vi "HEWH Pressure Calculation.vi"(9 "MW100 Data Cluster":T1) -> (1 "Pressure Adjusted":T1)   [LabVIEW 2019]
uses:
  Type Definitions/HEWH MW100 Data Cluster.ctl
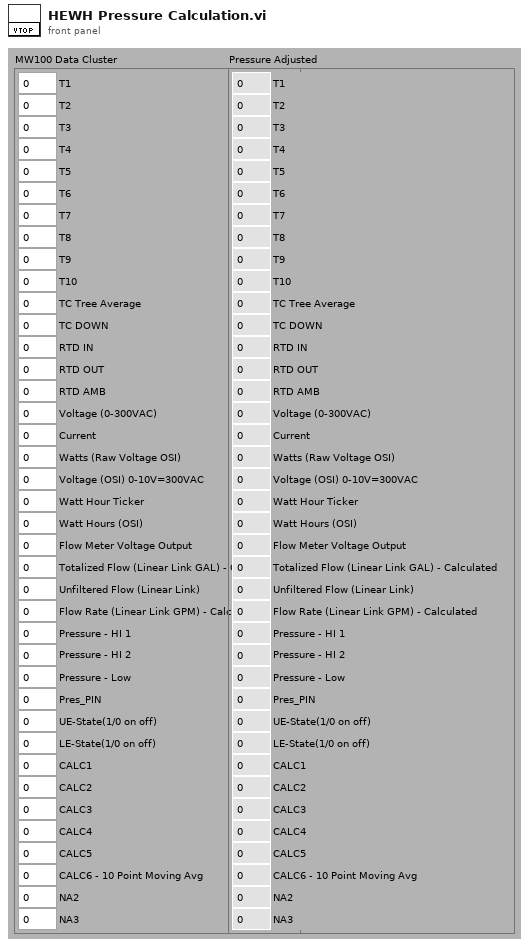
[diagram p1: front panel]
types:
  T1 = typedef "HEWH MW100 Data Cluster.ctl" = cluster{"T1":dbl, "T2":dbl, "T3":dbl, "T4":dbl, "T5":dbl, "T6":dbl, "T7":dbl, "T8":dbl, "T9":dbl, "T10":dbl, "TC Tree Average":dbl, "TC DOWN":dbl, "RTD IN":dbl, "RTD OUT":dbl, "RTD AMB":dbl, "Voltage (0-300VAC)":dbl, "Current":dbl, "Watts (Raw Voltage OSI)":dbl, "Voltage (OSI) 0-10V=300VAC":dbl, "Watt Hour Ticker":dbl, "Watt Hours (OSI)":dbl, "Flow Meter Voltage Output":dbl, "Totalized Flow (Linear Link GAL) - Calculated":dbl, "Unfiltered Flow (Linear Link)":dbl, "Flow Rate (Linear Link GPM) - Calculated":dbl, "Pressure - HI 1":dbl, "Pressure - HI 2":dbl, "Pressure - Low":dbl, "Pres_PIN":dbl, "UE-State(1/0 on off)":dbl, "LE-State(1/0 on off)":dbl, "CALC1":dbl, "CALC2":dbl, "CALC3":dbl, "CALC4":dbl, "CALC5":dbl, "CALC6 - 10 Point Moving Avg":dbl, "NA2":dbl, "NA3":dbl}
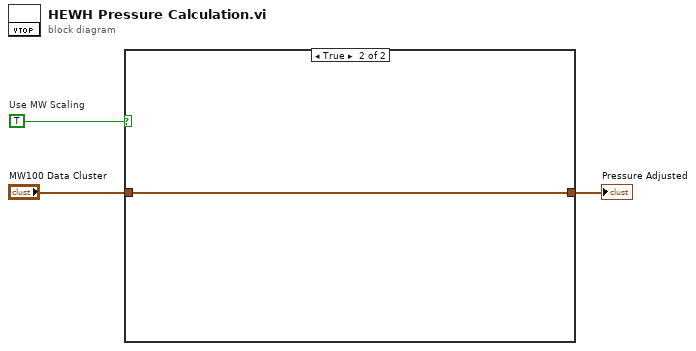
[diagram p0: block diagram]
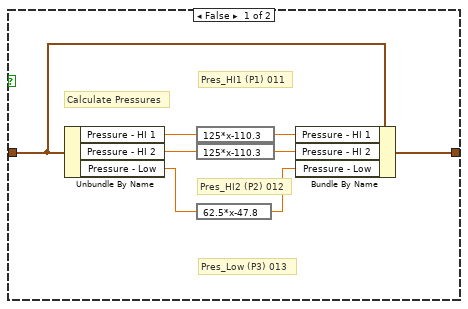
[diagram p2: hidden frame]
diagram:
  w1 = TRUE  # Use MW Scaling
  n1 = case shown="True" w1 {
    tunnel: "MW100 Data Cluster" -> [w8 w12]
    tunnel: [w4 w12] -> w2
    frame False {
      # "Pres_Low (P3) 013"
      # "Pres_HI2 (P2) 012"
      # "Pres_HI1 (P1) 011"
      # "Calculate Pressures"
      n2 = Unbundle By Name(w8) -> ("Pressure - HI 1"=w11:dbl, "Pressure - HI 2"=w10:dbl, "Pressure - Low"=w9:dbl)
      n3 = expression code="125*x-110.3"(w11) -> (w7:dbl)
      n4 = expression code="125*x-110.3"(w10) -> (w6:dbl)
      n5 = expression code="62.5*x-47.8"(w9) -> (w5:dbl)
      n6 = Bundle By Name(cluster=w8, "Pressure - HI 1"=w7, "Pressure - HI 2"=w6, "Pressure - Low"=w5) -> (w4:T1)
    }
    frame True {
    }
  }
  "Pressure Adjusted" <- w2
